vi "GenericDriveWriteMulti.vi"(1 "Channel Description":T3={"Channel Name"="", "Vel. Default"=5.0, "Acc. Default"=5.0, "Vel. Max"=5.0, "Vel. Min"=5.0, "Acc. Max"=5.0, "Acc. Min"=5.0, "Pulses/unit"=0.0, "Address"=0, "Pulse Offset"=0, "Pos Tolerance"=0.0, "Pulses/rev"=0.0, "Backlash/Eng units"=0.0, "Current Pos"=0.0, "Ch Status"=enum."Active", "Port Name"="", "Axis Transform mode"="", "Metadata Ch Name"="", "Type"=""} {"Current Pos" format="%.2f"; "Backlash/Eng units" format="%.2f"; "Pulses/rev" format="%.2f"; "Pos Tolerance" format="%.2f"; "Pulses/unit" format="%.2f"; "Acc. Min" format="%.2f"; "Acc. Max" format="%.2f"; "Vel. Min" format="%.2f"; "Vel. Max" format="%.2f"; "Acc. Default" format="%.2f"; "Vel. Default" format="%.2f"}, 2 "Array Constant":T2(array[cluster])=[{"GenericDriveCommand"="DePowerMotor", "Numeric Value"=0.0}, {"GenericDriveCommand"="DePowerMotor", "Numeric Value"=0.0}, {"GenericDriveCommand"="DePowerMotor", "Numeric Value"=0.0}] {"Numeric Value" format="%.2f"}) -> ()   [LabVIEW 2010]
uses:
  DriveProperties.ctl
  GenericDriveCommand.ctl
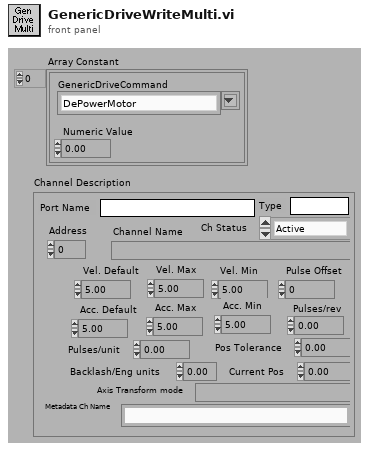
[diagram p1: front panel]
types:
  T1 = typedef "GenericDriveCommand.ctl" = string
  T2 = cluster{"GenericDriveCommand":T1, "Numeric Value":dbl}[]
  T3 = typedef "DriveProperties.ctl" = cluster{"Channel Name":string, "Vel. Default":dbl, "Acc. Default":dbl, "Vel. Max":dbl, "Vel. Min":dbl, "Acc. Max":dbl, "Acc. Min":dbl, "Pulses/unit":dbl, "Address":u8, "Pulse Offset":i32, "Pos Tolerance":dbl, "Pulses/rev":dbl, "Backlash/Eng units":dbl, "Current Pos":dbl, "Ch Status":enum16{"Active", "Offline", "Simulate"}, "Port Name":string, "Axis Transform mode":string, "Metadata Ch Name":string, "Type":string}
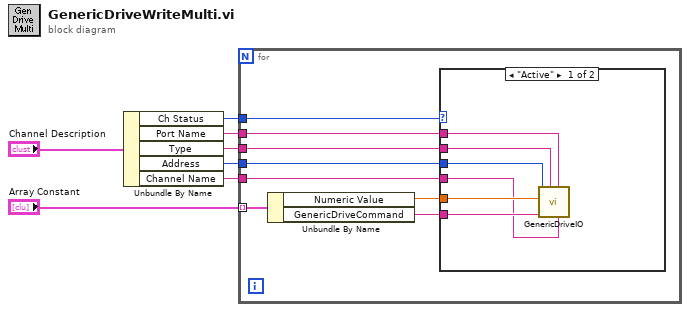
[diagram p0: block diagram]
diagram:
  n1 = Unbundle By Name("Channel Description") -> ("Ch Status"=w5:enum16{"Active", "Offline", "Simulate"}, "Port Name"=w4:string, "Type"=w3:string, "Address"=w2:u8, "Channel Name"=w1:string)
  n2 = for {
    tunnel: "Array Constant" -> [w15] mode=indexing
    tunnel: w5 -> [w14]
    tunnel: w4 -> [w13]
    tunnel: w3 -> [w12]
    tunnel: w2 -> [w11]
    tunnel: w1 -> [w8]
    n3 = Unbundle By Name(w15) -> ("Numeric Value"=w10:dbl, "GenericDriveCommand"=w9:T1)
    n4 = case shown="\"Active\"" w14 {
      tunnel: w13 -> [w21 _]
      tunnel: w12 -> [w20 _]
      tunnel: w11 -> [w19 _]
      tunnel: w10 -> [w18 _]
      tunnel: w9 -> [w17 _]
      tunnel: w8 -> [w16 _]
      frame "Active" {
        n5 = call "GenericDriveIO.vi"("GenericDriveCommand"=w17, "Channel Name"=w16, "Numeric Value"=w18, "Address"=w19, "Type"=w20, "Port Name"=w21) -> ()  [unwired: 1 in, 5 out]
      }
      frame "Offline", Default {
      }
    }
  }
